vi "Solve1.vi"(8 "Error In":errorcluster, 11 "object in":refnum<class "2021_8.lvclass">) -> (0 "Error Out":errorcluster, 2 "Result":u64, 3 "object out":refnum<class "2021_8.lvclass">)   [LabVIEW 2020, in "2021_8.lvclass"]
uses:
  2021_8.lvclass
  2021_8.lvclass/2021_8.ctl
  bc245b98-c824-4be9-8c29-8e4744b8ca36.vi
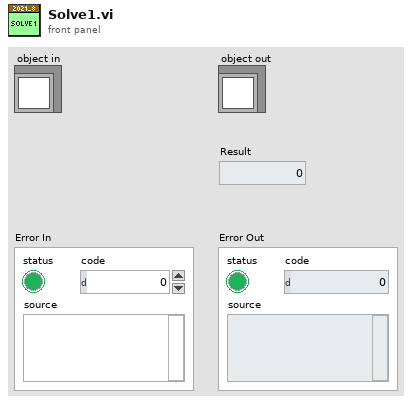
[diagram p1: front panel]
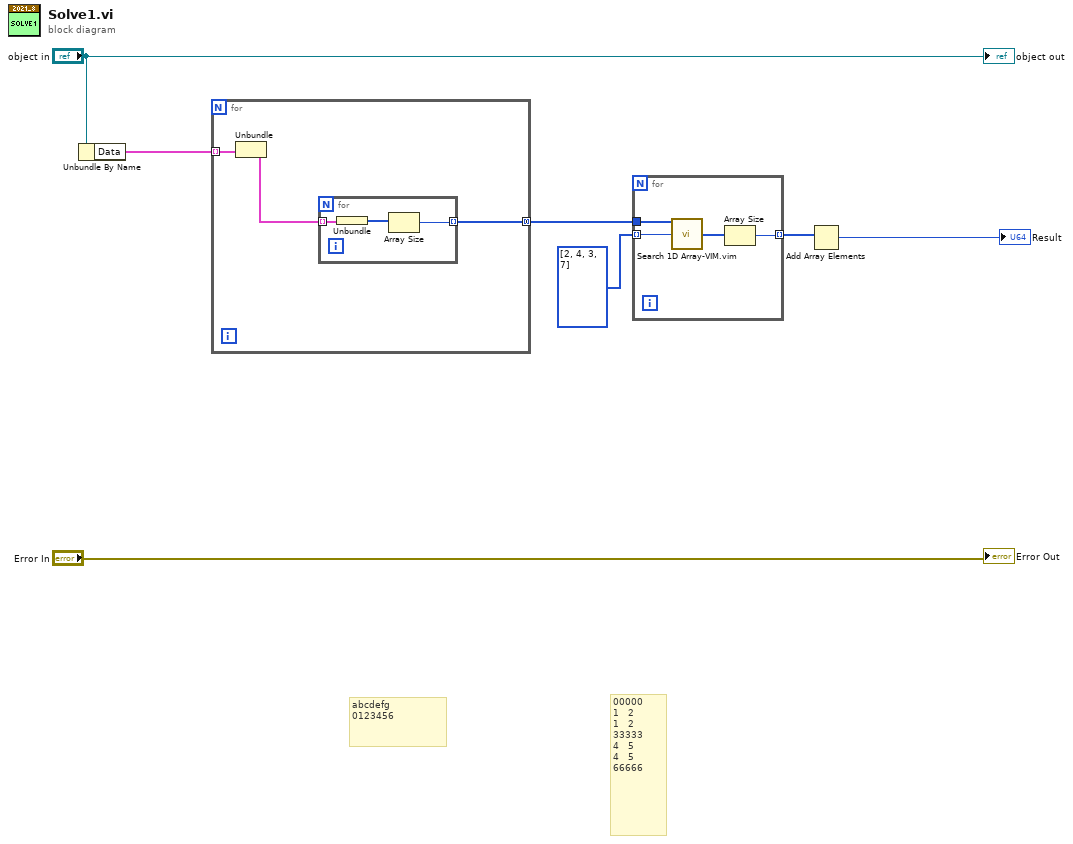
[diagram p0: block diagram]
diagram:
  # "00000\n1   2\n1   2\n33333\n4   5\n4   5\n66666"
  # "abcdefg\n0123456"
  n1 = Unbundle By Name("object in") -> ("Data"=w5:cluster{cluster{i32[]}[], cluster{i32[]}[]}[])
  n2 = for {
    tunnel: w5 -> [w10] mode=indexing
    tunnel: [w8] -> w4 mode=concatenating
    n3 = Unbundle(w10) -> (w9:cluster{i32[]}[])  [unwired: 1 out]
    n4 = for {
      tunnel: w9 -> [w13] mode=indexing
      tunnel: [w11] -> w8 mode=indexing
      n5 = Unbundle(w13) -> (w12:i32[])
      n6 = Array Size(array=w12) -> (size(s)=w11:i32)
    }
  }
  n7 = for {
    tunnel: w4 -> [w17]
    tunnel: i32[] [2, 4, 3, 7] -> [w16] mode=indexing
    tunnel: [w14] -> w2 mode=indexing
    n8 = call "Search 1D Array-VIM.vim"("Array"=w17, "Element Data"=w16) -> ("Indices of Elements"=w15:i32[])  [unwired: 7 in]
    n9 = Array Size(array=w15) -> (size(s)=w14:i32)
  }
  n10 = Add Array Elements(numeric array=w2) -> (sum=→"Result":i32)
  "Error Out" <- "Error In"
  "object out" <- "object in"
